vi "Output Configuration (Set).vi"(6 "ISOBUS address":T4=-1 caption="ISOBUS address (-1)", 8 "error in":errorcluster, 10 "Out Config":T1="SERS" caption="Output Configuration", 11 "Mercury Reference In":T5) -> (0 "error out":errorcluster, 2 "Response":T2, 3 "Mercury Reference Out":T5, 4 "Valid?":T3)   [LabVIEW 2016, in "Mercury iXX.lvlib" / "Magnet.lvlib"]
doc: "Set the output configuration.\n\nNB: The instrument must be in Engineering mode to set this item."
uses:
  Magnet.lvlib
  Controls/Mercury Reference.ctl
  Controls/Comms Transport Layer.ctl
  Private/Controls/Query Dynamic Reference.ctl
  Controls/ISOBus Address.ctl
  Controls/Is Valid LED.ctl
  Controls/Response String.ctl
  Controls/Output Configuration.ctl
  Private/Controls/Command Verbs.ctl
  Mercury iXX.lvlib
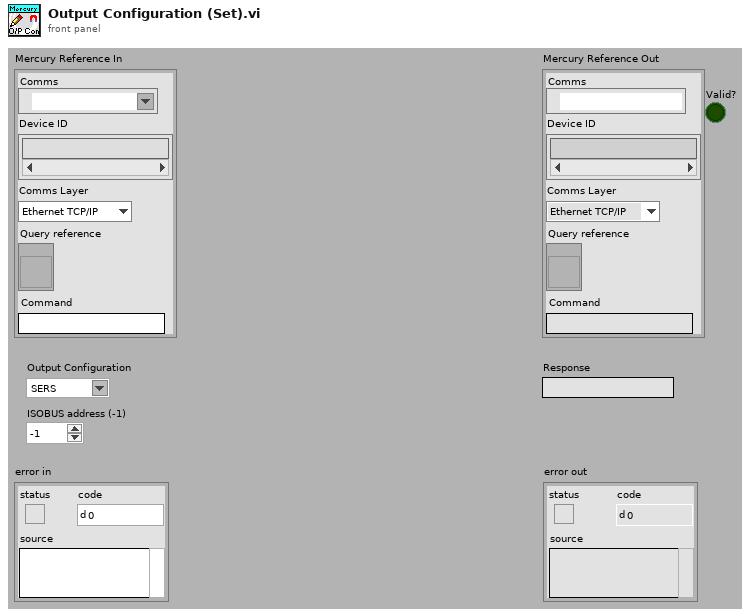
[diagram p1: front panel]
types:
  T1 = typedef "Mercury iXX.lvlib/Magnet.lvlib/Output Configuration.ctl" = string
  T2 = typedef "Mercury iXX.lvlib/Response String.ctl" = string
  T3 = typedef "Mercury iXX.lvlib/Is Valid LED.ctl" = bool
  T4 = typedef "Mercury iXX.lvlib/ISOBus Address.ctl" = i32
  T5 = typedef "Mercury iXX.lvlib/Mercury Reference.ctl" = cluster{"Comms":refnum<visa-resource-name>, "Device ID":string[], "Comms Layer":T6, "Command":string, "Query reference":T7}
  T6 = typedef "Mercury iXX.lvlib/Comms Transport Layer.ctl" = enum16{"Ethernet TCP/IP", "USB", "ISOBus - RS-232", "GPIB"}
  T7 = typedef "Mercury iXX.lvlib/Query Dynamic Reference.ctl" = refnum<vi>
  T8 = typedef "Mercury iXX.lvlib/Command Verbs.ctl" = string
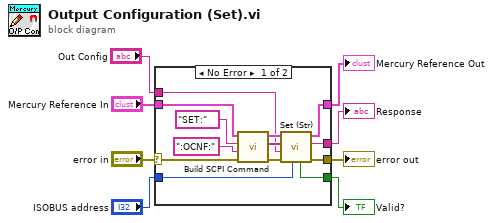
[diagram p0: block diagram]
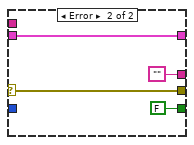
[diagram p2: hidden frame]
diagram:
  n1 = case shown="No Error" "error in" {
    selector: "error in" -> [w15 w24]
    tunnel: "Mercury Reference In" -> [w12 w25]
    tunnel: [w21 w24] -> w7
    tunnel: [w20 w25] -> w6
    tunnel: "ISOBUS address" -> [w19 _]
    tunnel: [w18 T3 FALSE ("Valid?")] -> w4
    tunnel: [w17 ""] -> w3
    tunnel: "Out Config" -> [w9 _]
    frame No Error {
      n2 = call "Build SCPI Command.vi"("error in"=w15, "Noun(s)"=":OCNF:" ("Command"), "Verb"=T8 "SET:", "Mercury Reference In"=w12) -> ("error out"=w16:errorcluster, "SCPI Message(s)"=w10:string[], "Mercury Reference Out"=w11:T5)  [unwired: 5 out]
      n3 = call "Set (Str).vi"("ISOBUS address"=w19, "error in"=w16, "Command Value (Str)"=w9, "SCPI Message(s)"=w10, "Mercury Reference In"=w11) -> ("error out"=w21:errorcluster, "Response"=w17:T2, "Mercury Reference Out"=w20:T5, "Valid?"=w18:T3)  [unwired: 3 out]
    }
    frame Error {
    }
  }
  "Mercury Reference Out" <- w6
  "error out" <- w7
  "Valid?" <- w4
  "Response" <- w3
